vi "ReplacePolySubVINode.vi"(5 "Old File Name":string="PolyA String.vi", 7 "New File Name":string="PolyB.vi", 8 "error in (no error)":errorcluster, 11 "VI Refnum":refnum<vi>) -> (0 "error out":errorcluster, 3 "VI Refnum Out":refnum<vi>, 4 "Replaced":bool)   [LabVIEW 2024]
uses:
  <vilib>/Utility/traverseref.llb/TRef TravTarget.ctl
  <vilib>/Utility/traverseref.llb/VI Scripting - Traverse.lvlib
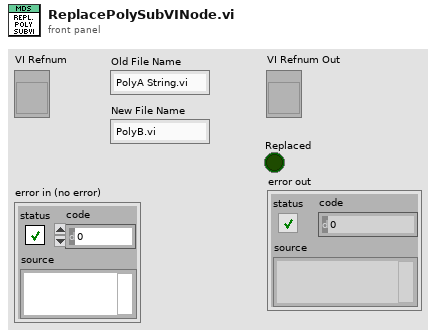
[diagram p1: front panel]
types:
  T1 = typedef "TRef TravTarget.ctl" = enum16{"FP", "BD", "Other"}
  T2 = cluster{"VIPath":path, "Menu Name":string, "Selector Name":string}[]
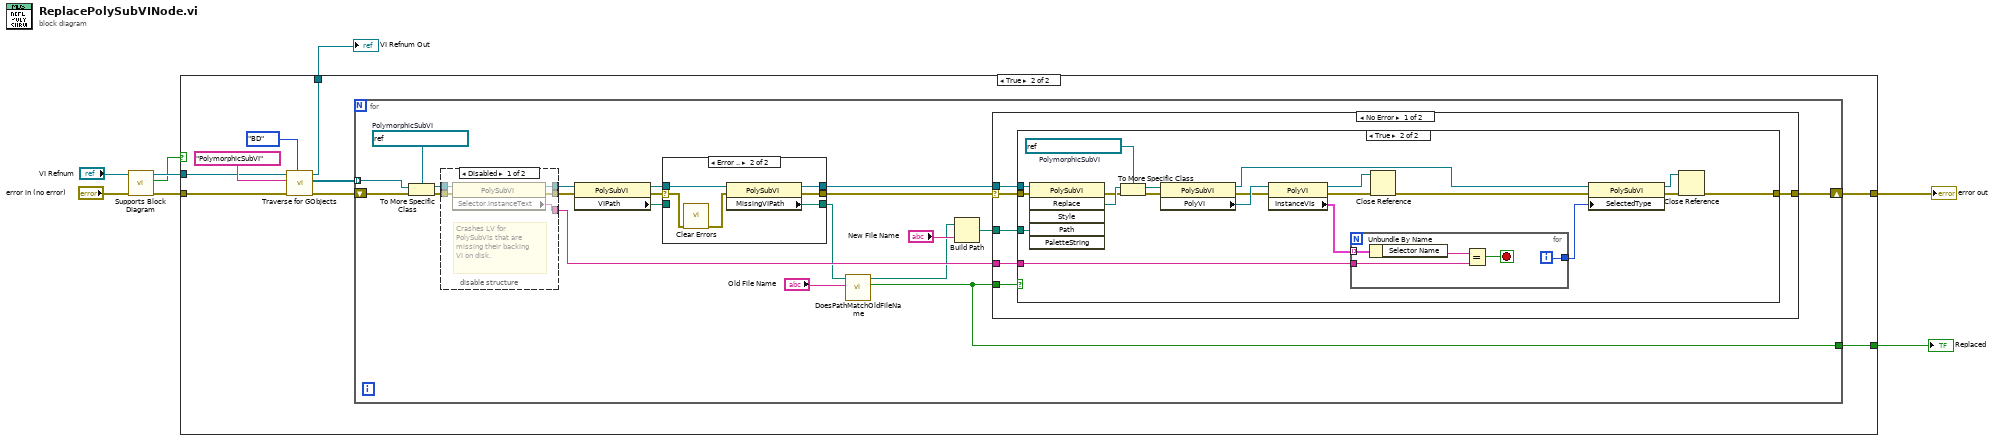
[diagram p0: block diagram]
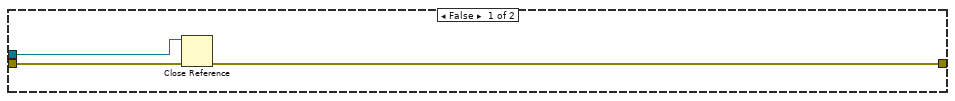
[diagram p3: hidden frame]
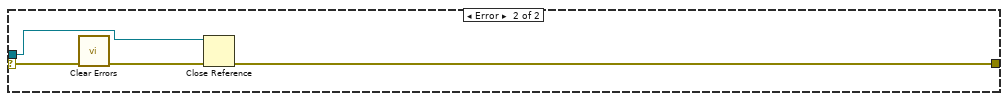
[diagram p4: hidden frame]
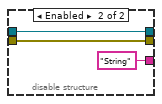
[diagram p5: hidden frame]
diagram:
  n1 = call "Supports Block Diagram.vi"("error in (no error)"="error in (no error)", "vi in"="VI Refnum") -> ("error out"=w3:errorcluster, "has block diagram"=w1:bool, "vi out"=w4:refnum<vi>)  [unwired: 7 in]
  n2 = case shown="True" w1 {
    tunnel: [_ w15] -> w8
    tunnel: [w9 w14] -> w7
    tunnel: w4 -> [w10 w13]
    tunnel: w3 -> [w9 w12]
    tunnel: [w10 w11] -> w6
    frame False {
    }
    frame True {
      n3 = call <vilib>:"Traverse for GObjects.vi"("Traverse Target"=TRef_TravTarget."BD", "error in (no error)"=w12, "Class Name"="PolymorphicSubVI", "VI Refnum"=w13) -> ("error out"=w18:errorcluster, "References"=w19:refnum<vi>[], "dup VI Refnum"=w11:refnum<vi>)  [unwired: 4 in, 1 out]
      n4 = for {
        shift-right: [w33] -> w14
        shift-left: w18 -> [w37]
        tunnel: w19 -> [w38] mode=indexing
        tunnel: [w21] -> w15
        w39 = refnum<vi> refnum  # PolymorphicSubVI
        n5 = To More Specific Class(target class=w39, reference=w38, error in=w37) -> (specific class reference=w28:refnum<vi>, error out=w26:errorcluster)
        n6 = disable-structure shown="Disabled" {
          disable-tunnel: w28 -> [w82 w85]
          disable-tunnel: [w81 w85] -> w27
          disable-tunnel: w26 -> [w80 w84]
          disable-tunnel: [w79 w84] -> w25
          disable-tunnel: [w78 "String" ("Selector.InstanceText")] -> w24
          frame Disabled {
            # "Crashes LV for PolySubVIs that are missing their backing VI on disk."
            n7 = property class="PolySubVI"(reference=w82, error in=w80) -> (reference out=w81:refnum<vi>, error out=w79:errorcluster, "Selector.InstanceText"=w78:string)
          }
          frame Enabled {
          }
        }
        n8 = property class="PolySubVI"(reference=w27, error in=w25) -> (reference out=w35:refnum<vi>, error out=w34:errorcluster, "VIPath"=w36:path)
        n9 = case shown="Error .." w34 {
          selector: w34 -> [w88 w94]
          tunnel: w36 -> [w87 _]
          tunnel: [w88 w92] -> w31
          tunnel: w35 -> [w86 w91]
          tunnel: [w86 w90] -> w32
          tunnel: [w87 w89] -> w23
          frame No Error {
          }
          frame Error {
            n10 = call <vilib>:"Clear Errors.vi"("error in (no error)"=w94) -> ("error out"=w93:errorcluster)  [unwired: 5 in, 1 out]
            n11 = property class="PolySubVI"(reference=w91, error in=w93) -> (reference out=w90:refnum<vi>, error out=w92:errorcluster, "MissingVIPath"=w89:path)
          }
        }
        n12 = call "DoesPathMatchOldFileName.vi"("Old File Name"="Old File Name", "File Path"=w23) -> ("Match Found"=w21:bool, "Parent Directory"=w20:path)  [unwired: 8 in]
        n13 = Build Path(base path=w20, name or relative path="New File Name") -> (appended path=w29:path)
        n14 = case shown="No Error" w31 {
          selector: w31 -> [w41 w77]
          tunnel: w29 -> [w45 _]
          tunnel: w21 -> [w44 _]
          tunnel: [w43 w74] -> w33
          tunnel: w32 -> [w42 w75]
          tunnel: w24 -> [w40 _]
          frame No Error {
            n15 = case shown="True" w44 {
              tunnel: w45 -> [_ w68]
              tunnel: w41 -> [w48 w67]
              tunnel: [w47 w49] -> w43
              tunnel: w42 -> [w46 w66]
              tunnel: w40 -> [_ w58]
              frame False {
                n16 = Close Reference(reference=w46, error in (no error)=w48) -> (error out=w47:errorcluster)
              }
              frame True {
                w64 = refnum<vi> refnum  # PolymorphicSubVI
                n17 = invoke class="PolySubVI" method="Replace"(reference=w66, error in=w67, "Path"=w68) -> (error out=w63:errorcluster, "Replace"=w65:refnum<vi>)  [unwired: 3 in, 4 out]
                n18 = To More Specific Class(target class=w64, reference=w65, error in=w63) -> (specific class reference=w61:refnum<vi>, error out=w62:errorcluster)
                n19 = property class="PolySubVI"(reference=w61, error in=w62) -> (reference out=w56:refnum<vi>, error out=w57:errorcluster, "PolyVI"=w60:refnum<vi>)
                n20 = property class="PolyVI"(reference=w60, error in=w57) -> (reference out=w52:refnum<vi>, error out=w54:errorcluster, "InstanceVIs"=w59:T2)
                n21 = for {
                  tunnel: w59 -> [w72] mode=indexing
                  tunnel: w58 -> [w73]
                  tunnel: [w69] -> w55
                  i -> [w69]
                  stop <- w70 stop-if-true
                  n22 = Unbundle By Name(w72) -> ("Selector Name"=w71:string)
                  n23 = Equal?(x=w71, y=w73) -> (x = y?=w70:bool)
                }
                n24 = Close Reference(reference=w52, error in (no error)=w54) -> (error out=w53:errorcluster)
                n25 = property class="PolySubVI"(reference=w56, error in=w53, "SelectedType"=w55) -> (reference out=w50:refnum<vi>, error out=w51:errorcluster)
                n26 = Close Reference(reference=w50, error in (no error)=w51) -> (error out=w49:errorcluster)
              }
            }
          }
          frame Error {
            n27 = call <vilib>:"Clear Errors.vi"("error in (no error)"=w77) -> ("error out"=w76:errorcluster)  [unwired: 5 in, 1 out]
            n28 = Close Reference(reference=w75, error in (no error)=w76) -> (error out=w74:errorcluster)
          }
        }
      }
    }
  }
  "error out" <- w7
  "Replaced" <- w8
  "VI Refnum Out" <- w6
